vi "System Definition To Parameters.vi"(8 "error in":errorcluster, 10 "direction":T2, 11 "label ref":T5 format="%.0x") -> (0 "error out":errorcluster, 2 "parameters":T1[](array[typedef]), 3 "label ref out":T5 format="%.0x")   [LabVIEW 2020, in "Ballard ARINC 429 Scripting.lvlib"]
uses:
  Ballard ARINC 429 Scripting.lvlib
  Encoding and Decoding/Encoding.ctl
  Encoding and Decoding/Encoding and Decoding.lvlib
  Shared/Parameter Definition.ctl
  Shared/Direction.ctl
  Shared/VS Channel Definition for Parameter.ctl
  ARINC 429/ARINC 429 Scripting.lvlib
  <vilib>/NI VeriStand/Custom Device API/Custom Device Item Ref.ctl
  <vilib>/NI VeriStand/Custom Device API/Custom Device API.lvlib
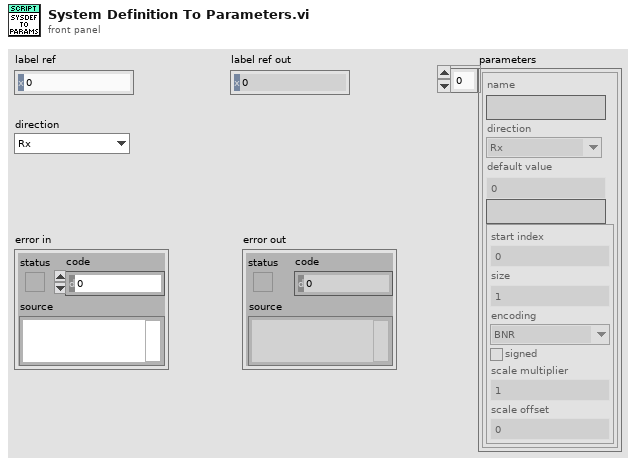
[diagram p1: front panel]
types:
  T1 = typedef "VS Channel Definition for Parameter.ctl" = cluster{"name":string, "direction":T2, "default value":dbl, "unit":string, "Parameter":T3}
  T2 = typedef "Direction.ctl" = enum16{"Rx", "Tx"}
  T3 = typedef "Parameter Definition.ctl" = cluster{"start index":i32, "size":i32, "encoding":T4, "signed":bool, "scale multiplier":dbl, "scale offset":dbl}
  T4 = typedef "Encoding and Decoding.lvlib/Encoding.ctl" = enum16{"BNR", "BCD", "Discrete"}
  T5 = typedef "Custom Device API.lvlib/Custom Device Item Ref.ctl" = u64
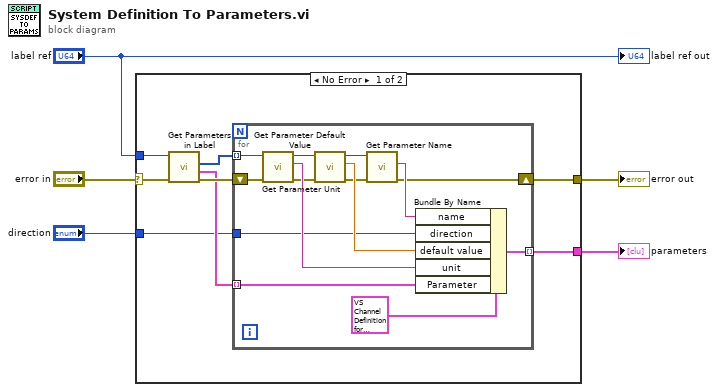
[diagram p0: block diagram]
diagram:
  n1 = case shown="No Error" "error in" {
    selector: "error in" -> [w8 w28]
    tunnel: "label ref" -> [w6 _]
    tunnel: [w10 w28] -> w5
    tunnel: [w9 _] -> w2
    tunnel: "direction" -> [w7 _]
    frame No Error {
      n2 = call "Get Parameters in Label.vi"("error in"=w8, "label ref"=w6) -> ("error out"=w13:errorcluster, "parameter definitions"=w12:T3[], "parameter references"=w11:T5[])  [unwired: 6 in, 1 out]
      n3 = for {
        shift-right: [w15] -> w10
        shift-left: w13 -> [w24]
        tunnel: w12 -> [w26] mode=indexing
        tunnel: [w25] -> w9 mode=indexing
        tunnel: w11 -> [w23] mode=indexing
        tunnel: w7 -> [w14]
        n4 = call "Get Parameter Unit.vi"("error in"=w24, "parameter ref"=w23) -> ("error out"=w21:errorcluster, "unit"=w22:string, "parameter ref out"=w20:T5)  [unwired: 7 in]
        n5 = call "Get Parameter Default Value.vi"("error in"=w21, "parameter ref"=w20) -> ("error out"=w18:errorcluster, "Default Value (Scaled)"=w19:dbl, "parameter ref out"=w17:T5)  [unwired: 7 in]
        n6 = call "Get Parameter Name.vi"("error in"=w18, "parameter ref"=w17) -> ("error out"=w15:errorcluster, "name"=w16:string)  [unwired: 7 in, 1 out]
        n7 = Bundle By Name(cluster=T1 {"name"="", "direction"=enum."Rx", "default value"=0.0, "unit"="", "Parameter"={"start index"=0, "size"=1, "encoding"=enum."BNR", "signed"=FALSE, "scale multiplier"=1.0, "scale offset"=0.0}} ("channel parameter"), "name"=w16, "direction"=w14, "default value"=w19, "unit"=w22, "Parameter"=w26) -> (w25:T1)
      }
    }
    frame Error {
    }
  }
  "error out" <- w5
  "parameters" <- w2
  "label ref out" <- "label ref"
